vi "TemperatureLogger.vi"() -> ()   [LabVIEW 2022 SP3]
uses:
  <extravilib>/ChannelInstances/Tag-c(c(ref(LVObjVI()),bool),bool,bool,bool,path,u32,ref(UserDefinedRefnumTag))/Read With Abort.vi
  <extravilib>/ChannelInstances/Tag-c(c(ref(LVObjVI()),bool),bool,bool,bool,path,u32,ref(UserDefinedRefnumTag))/Write With Abort.vi
  <extravilib>/ChannelInstances/Tag-c(c(ref(LVObjVI()),bool),bool,bool,bool,path,u32,ref(UserDefinedRefnumTag))/Instantiate.vi
  <extravilib>/ChannelInstances/Tag-c(c(ref(LVObjVI()),bool),bool,bool,bool,path,u32,ref(UserDefinedRefnumTag))/EndpointRead.vi
  <vilib>/DAQmx/create/channels.llb/DAQmx Create Channel (AI-Temperature-Thermocouple).vi
  <extravilib>/ChannelInstances/Tag-c(c(ref(LVObjVI()),bool),bool,bool,bool,path,u32,ref(UserDefinedRefnumTag))/Endpoint.vi
  <extravilib>/ChannelInstances/Tag-c(c(ref(LVObjVI()),bool),bool,bool,bool,path,u32,ref(UserDefinedRefnumTag)).lvlib
panel:
  in  "NI Channel":tag
  in  "DAQmx Task":refnum<k21>
  in  "Thermc. Type":enum16{"J", "K", "N", "R", "S", "T", "B", "E"}(ring)
  in  "Start":bool
  out "Temperatures":dbl[][](graph)=[[1.25, 2.5, 3.7, 4.9], [1.25, 2.5, 3.7, 4.9], [1.25, 2.5, 3.7, 4.9], [1.25, 2.5, 3.7, 4.9], [1.25, 2.5, 3.7, 4.9], [1.25, 2.5, 3.7, 4.9], [1.25, 2.5, 3.7, 4.9], [1.25, 2.5, 3.7, 4.9], [1.25, 2.5, 3.7, 4.9], [1.25, 2.5, 3.7, 4.9], [1.25, 2.5, 3.7, 4.9], [1.25, 2.5, 3.7, 4.9], [1.25, 2.5, 3.7, 4.9], [1.25, 2.5, 3.7, 4.9], [1.25, 2.5, 3.7, 4.9], [1.25, 2.5, 3.7, 4.9], [1.25, 2.5, 3.7, 4.9], [1.25, 2.5, 3.7, 4.9], [1.25, 2.5, 3.7, 4.9], [1.25, 2.5, 3.7, 4.9], [1.25, 2.5, 3.7, 4.9], [1.25, 2.5, 3.7, 4.9], [1.25, 2.5, 3.7, 4.9], [1.25, 2.5, 3.7, 4.9], [1.25, 2.5, 3.7, 4.9], [1.25, 2.5, 3.7, 4.9], [1.25, 2.5, 3.7, 4.9], [1.25, 2.5, 3.7, 4.9], [1.25, 2.5, 3.7, 4.9], [1.25, 2.5, 3.7, 4.9], [1.25, 2.5, 3.7, 4.9], [1.25, 2.5, 3.7, 4.9], [1.25, 2.5, 3.7, 4.9], [1.25, 2.5, 3.7, 4.9], [1.25, 2.5, 3.7, 4.9], [1.25, 2.5, 3.7, 4.9], [1.25, 2.5, 3.7, 4.9], [1.25, 2.5, 3.7, 4.9], [1.25, 2.5, 3.7, 4.9], [1.25, 2.5, 3.7, 4.9], [1.25, 2.5, 3.7, 4.9], [1.25, 2.5, 3.7, 4.9], [1.25, 2.5, 3.7, 4.9], [1.25, 2.5, 3.7, 4.9], [1.25, 2.5, 3.7, 4.9], [1.25, 2.5, 3.7, 4.9], [1.25, 2.5, 3.7, 4.9], [1.25, 2.5, 3.7, 4.9]]
  out "String":string="Exiting"
  # "DAQmx Setup"
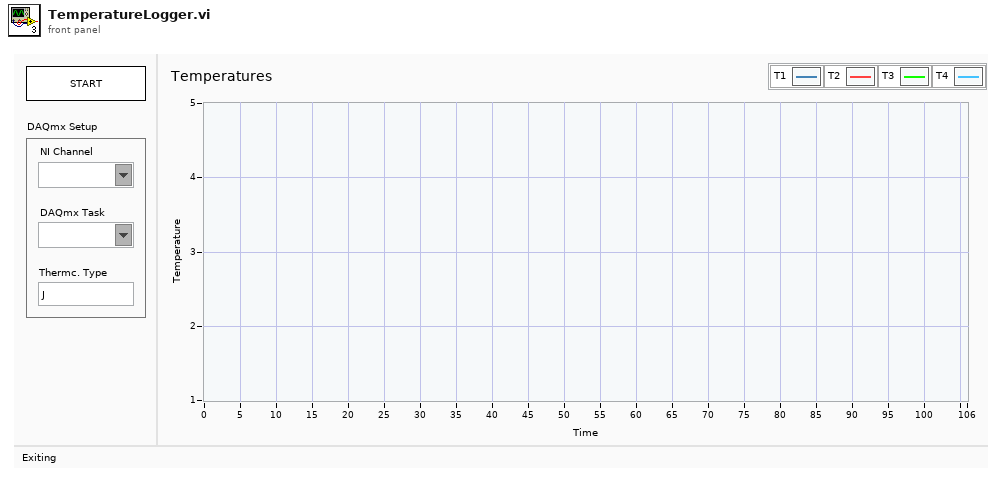
[diagram p1: front panel]
types:
  T1 = enum32{"Invalid", "Standard", "Closed", "Hidden", "Minimized", "Maximized"}
  T2 = enum32{"invalid app kind", "Development System", "Run Time System", "Student Edition", "Embedded LabVIEW", "Evaluation", "Custom"}
  T3 = cluster{"Core":cluster{"Current VI Reference":refnum<vi>, "Close Panel on Exit?":bool}, "System Active":bool, "Exit System":bool, "Connected":bool, "Data Path":path, "StartTime":u32, "NI Task":refnum<k21>}
  T4 = cluster{"Current VI Reference":refnum<vi>, "Close Panel on Exit?":bool}
  T5 = typedef "Tag-c(c(ref(LVObjVI()),bool),bool,bool,bool,path,u32,ref(UserDefinedRefnumTag)).lvlib/))Channel.ctl" = refnum<queue>
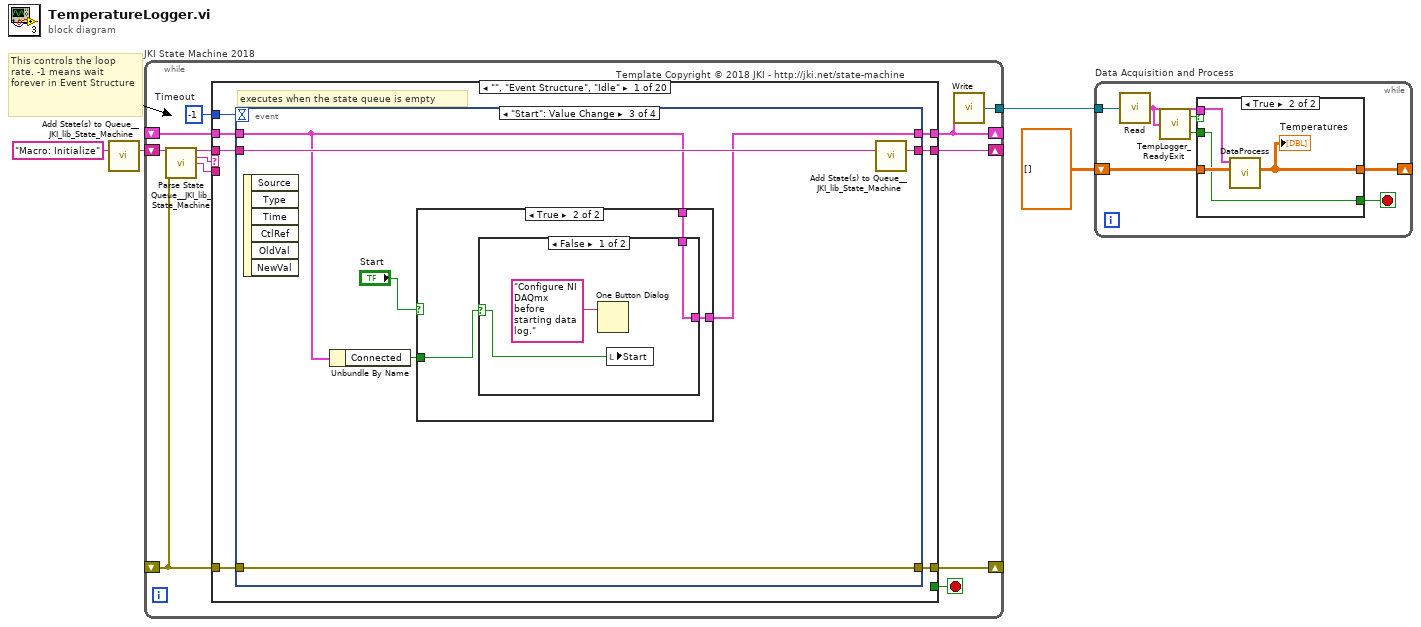
[diagram p0: block diagram]
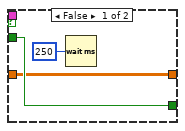
[diagram p2: hidden frame]
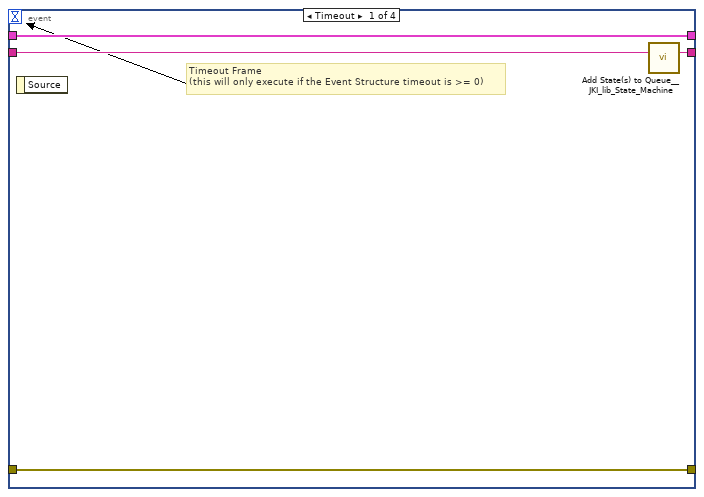
[diagram p3: hidden frame]
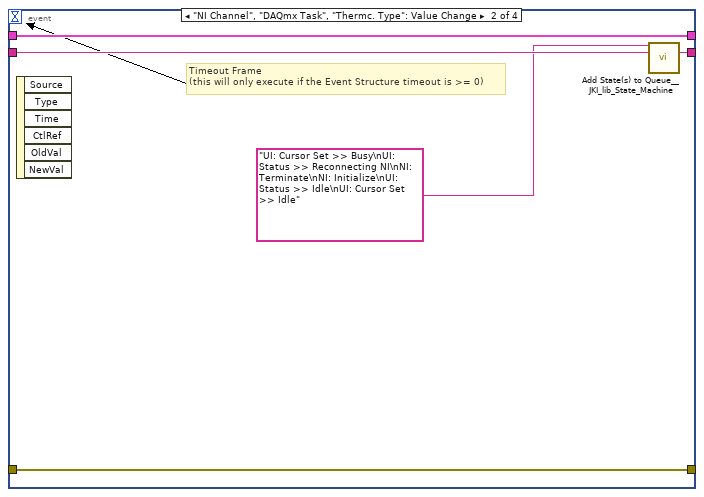
[diagram p4: hidden frame]
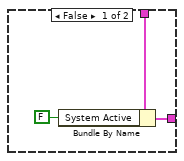
[diagram p5: hidden frame]
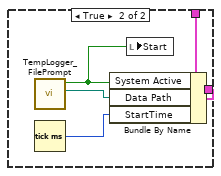
[diagram p6: hidden frame]
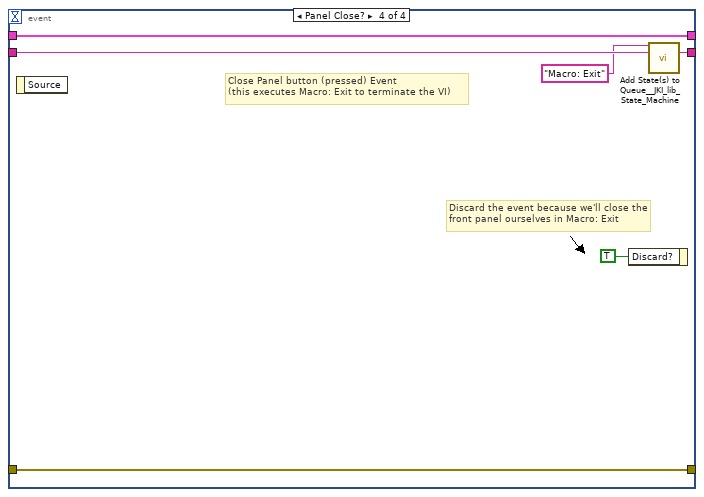
[diagram p7: hidden frame]
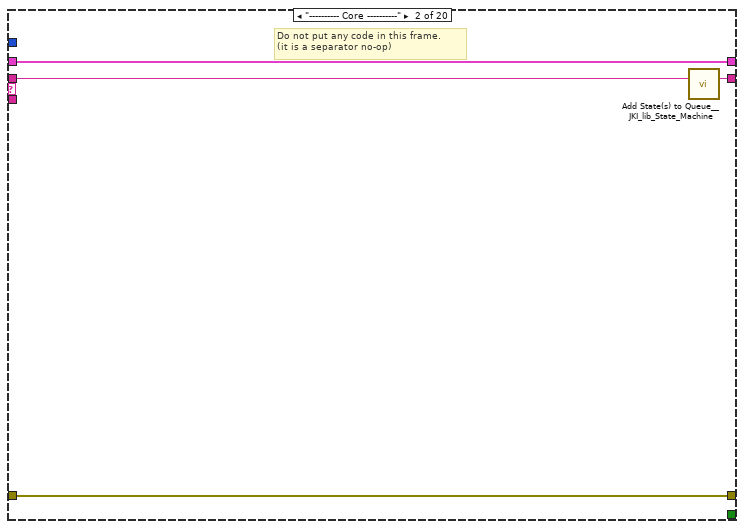
[diagram p8: hidden frame]
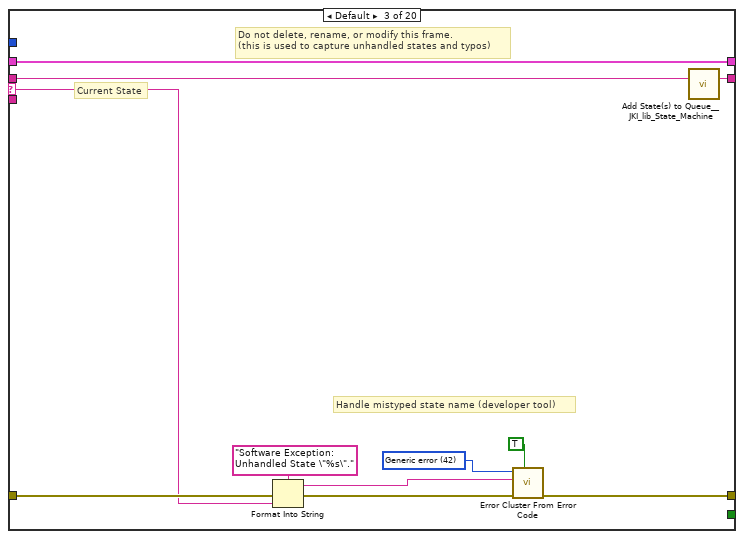
[diagram p9: hidden frame]
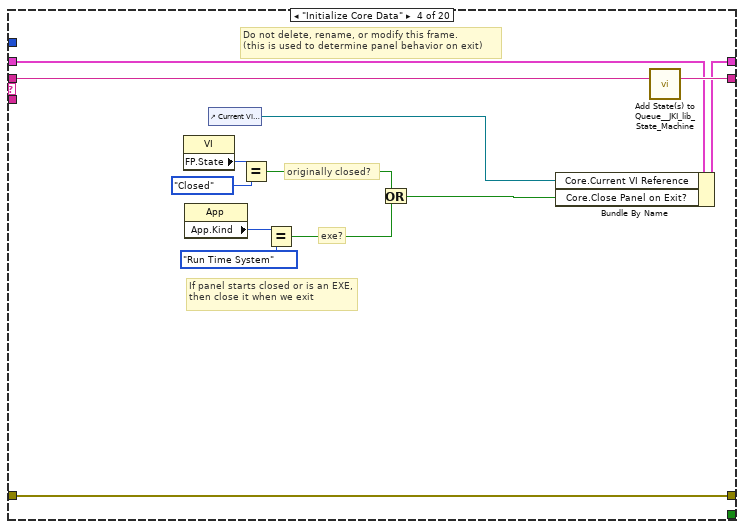
[diagram p10: hidden frame]
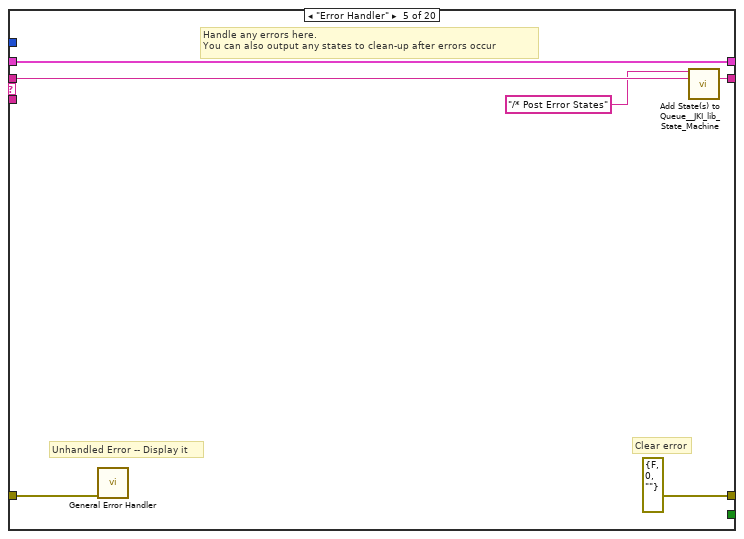
[diagram p11: hidden frame]
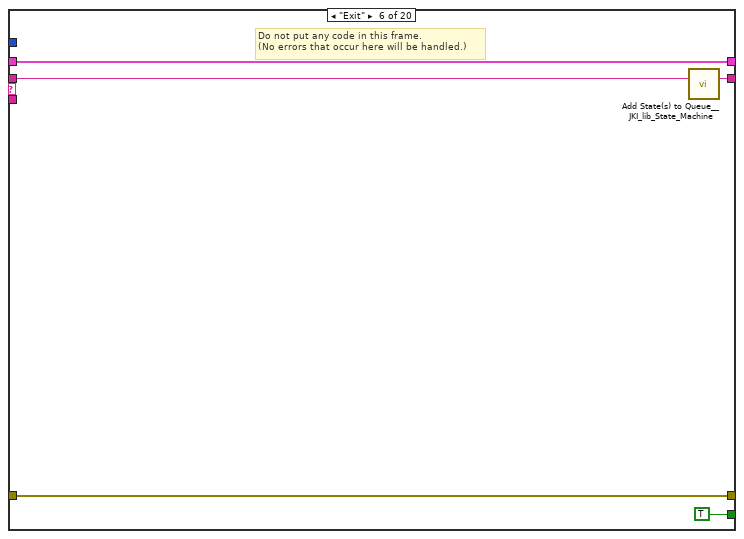
[diagram p12: hidden frame]
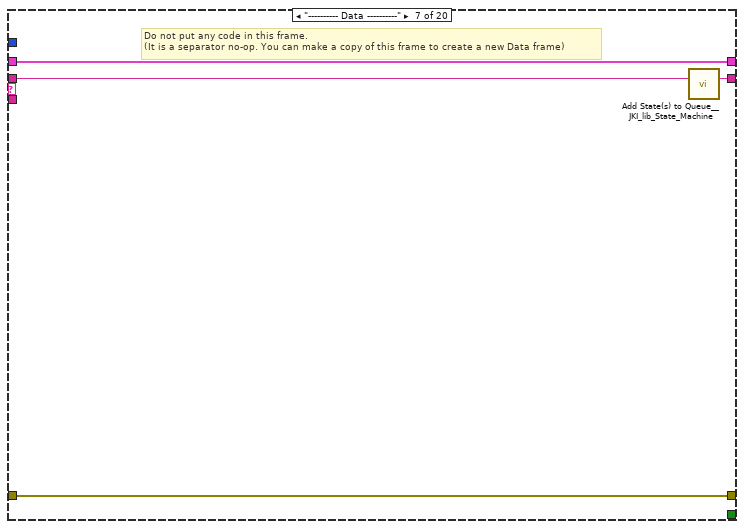
[diagram p13: hidden frame]
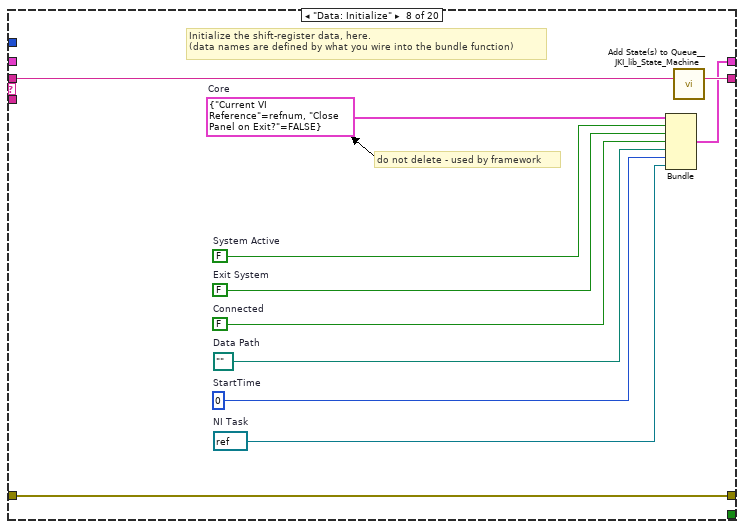
[diagram p14: hidden frame]
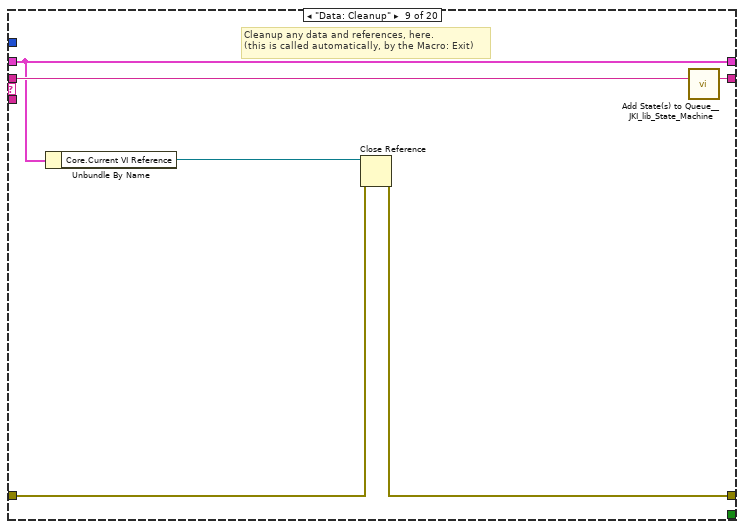
[diagram p15: hidden frame]
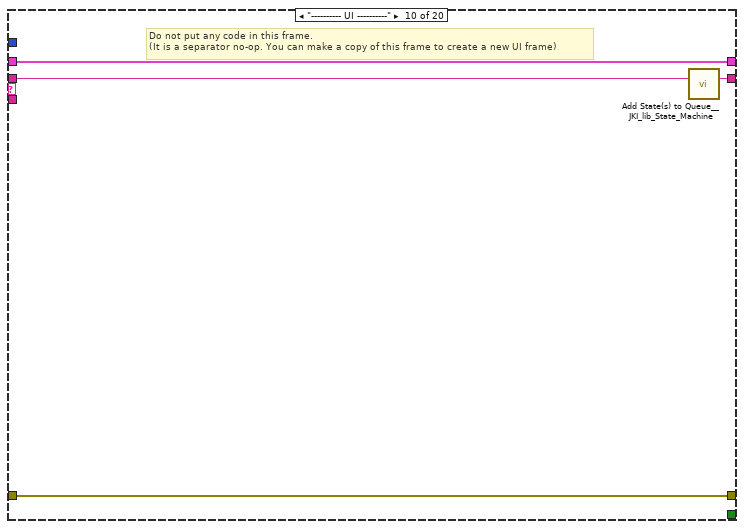
[diagram p16: hidden frame]
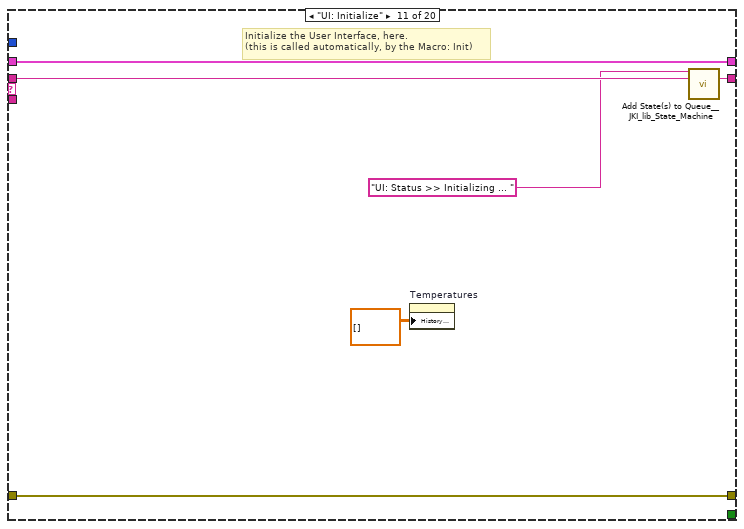
[diagram p17: hidden frame]
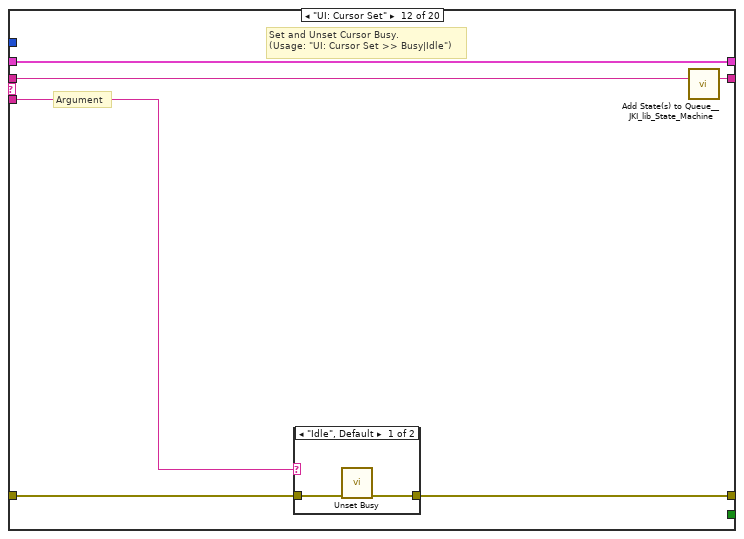
[diagram p18: hidden frame]
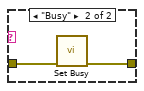
[diagram p19: hidden frame]
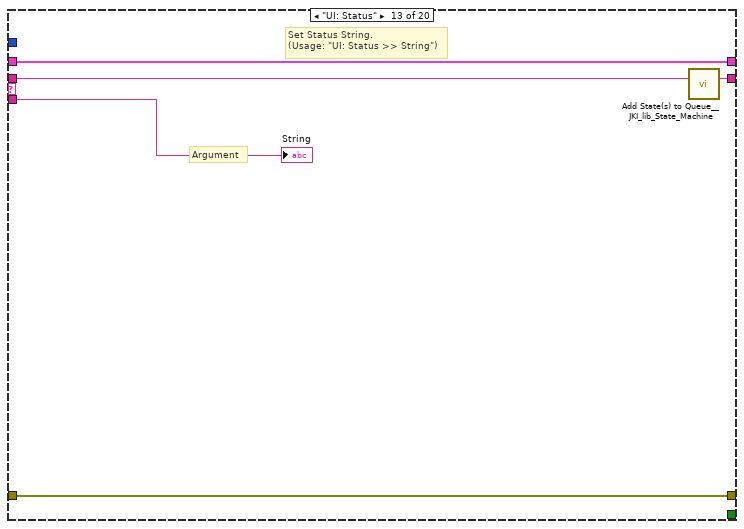
[diagram p20: hidden frame]
diagram:
  # "This controls the loop rate. -1 means wait forever in Event Structure"
  n1 = call <vilib>:"Add State(s) to Queue__JKI_lib_State_Machine.vi"("State(s) in (\"\")"="Macro: Initialize") -> ("States Out"=w4:string)  [unwired: 14 in]
  n2 = while "JKI State Machine 2018" {
    shift-right: [w6] -> _
    shift-left: _ -> [w9]
    shift-right: [w12] -> _
    shift-left: _ -> [w7]
    shift-right: [w11] -> _
    shift-left: w4 -> [w13]
    tunnel: [w5] -> w1
    stop <- w10 stop-if-true
    w8 = -1  # Timeout
    # "Template Copyright © 2018 JKI - http://jki.net/state-machine"
    n3 = call <vilib>:"Parse State Queue__JKI_lib_State_Machine.vi"("State Queue"=w13, "Error In (no error)"=w7) -> ("Remaining States"=w15:string, "Current State"=w16:string, "Arguments"=w14:string)  [unwired: 11 in]
    n4 = case shown="\"\", \"Event Structure\", \"Idle\"" w16 {
      selector: w16 -> [_ _ w64 _ _ _ _ _ _ _ _ _ _ _ _ _ _ _ _ _]
      tunnel: w15 -> [w23 w63 w68 w87 w93 w98 w102 w113 w119 w123 w129 w135 w144 w151 w220 w225 w237 w241 w253 w266]
      tunnel: w14 -> [_ _ _ _ _ _ _ _ _ _ _ w130 w141 w145 _ _ _ _ _ _]
      tunnel: w9 -> [w21 w60 w66 w80 w90 w96 w99 _ w114 w120 w127 w133 w142 w147 w217 w222 w234 w238 w250 w263]
      tunnel: [w20 w61 w70 w84 errorcluster {"status"=FALSE, "code"=0, "source"=""} ("error out") w95 w100 w110 w115 w121 w126 w131 w140 w148 w218 w223 w235 w239 w251 w264] -> w12
      tunnel: w7 -> [w19 w61 w69 w84 w89 w95 w100 w110 w116 w121 w126 w132 w140 w149 w218 w223 w235 w239 w251 w264]
      tunnel: [w22 w62 w67 w86 w92 w97 w101 w112 w118 w122 w128 w134 w143 w150 w219 w224 w236 w240 w252 w265] -> w11
      tunnel: [_ _ _ _ _ TRUE _ _ _ _ _ _ _ _ _ _ _ _ _ _] -> w10
      tunnel: [w18 w60 w66 w85 w90 w96 w99 w111 w114 w120 w127 w133 w142 w147 w217 w222 w227 w238 w244 w263] -> w6
      tunnel: w8 -> [w17 _ _ _ _ _ _ _ _ _ _ _ _ _ _ _ _ _ _ _]
      frame "", "Event Structure", "Idle" {
        # "executes when the state queue is empty"
        n5 = event shown="[2] \"Start\": Value Change" {
          selector: _ -> [_ _ _ _]
          dyn-events: _ -> [_ _ _ _]
          timeout: w17 -> [_ _ _ _]
          tunnel: w23 -> [w27 w32 w39 w59]
          tunnel: [w26 w31 w38 w58] -> w22
          tunnel: w21 -> [w24 w29 w34 w56]
          tunnel: [w25 w30 w37 w57] -> w20
          tunnel: w19 -> [w25 w30 w37 w57]
          tunnel: [w24 w29 w35 w56] -> w18
          event Timeout {
            # "Timeout Frame\n(this will only execute if the Event Structure timeout is >= 0)"
            n6 = event-data() -> ()  [unwired: 1 in, 1 out]
            n7 = call <vilib>:"Add State(s) to Queue__JKI_lib_State_Machine.vi"("State(s) in (\"\")"=w27) -> ("States Out"=w26:string)  [unwired: 14 in]
          }
          event "NI Channel", "DAQmx Task", "Thermc. Type": Value Change {
            # "Timeout Frame\n(this will only execute if the Event Structure timeout is >= 0)"
            n8 = event-data() -> ()  [unwired: 1 in, 6 out]
            n9 = call <vilib>:"Add State(s) to Queue__JKI_lib_State_Machine.vi"("State(s) in Front (\"\")"="UI: Cursor Set >> Busy\nUI: Status >> Reconnecting NI\nNI: Terminate\nNI: Initialize\nUI: Status >> Idle\nUI: Cursor Set >> Idle" ("State(s) in Front (\"\")"), "State(s) in (\"\")"=w32) -> ("States Out"=w31:string)  [unwired: 13 in]
          }
          event "Start": Value Change {
            n10 = event-data() -> ()  [unwired: 1 in, 6 out]
            n11 = Unbundle By Name(w34) -> ("Connected"=w33:bool)
            n12 = case shown="True" "Start" {
              tunnel: w34 -> [w40 w45]
              tunnel: [w41 w44] -> w35
              tunnel: w33 -> [_ w43]
              frame False {
                n13 = Bundle By Name(cluster=w40, "System Active"=FALSE) -> (w41:T3)
              }
              frame True {
                n14 = case shown="False" w43 {
                  selector: w43 -> [w46 _]
                  tunnel: w45 -> [w47 w53]
                  tunnel: [w47 w52] -> w44
                  frame False {
                    n15 = One Button Dialog(message="Configure NI DAQmx before starting data log.") -> ()  [unwired: 1 in, 1 out]
                    n16 = local write "Start"(w46) -> ()
                  }
                  frame True {
                    n17 = call "TempLogger_FilePrompt.vi"() -> ("selected path"=w51:path, "not cancelled"=w50:bool)  [unwired: 10 in]
                    n18 = Tick Count (ms)() -> (millisecond timer value=w49:u32)
                    n19 = Bundle By Name(cluster=w53, "System Active"=w50, "Data Path"=w51, "StartTime"=w49) -> (w52:T3)
                    n20 = local write "Start"(w50) -> ()
                  }
                }
              }
            }
            n21 = call <vilib>:"Add State(s) to Queue__JKI_lib_State_Machine.vi"("State(s) in (\"\")"=w39) -> ("States Out"=w38:string)  [unwired: 14 in]
          }
          event Panel Close? {
            # "Discard the event because we'll close the front panel ourselves in Macro: Exit"
            # "Close Panel button (pressed) Event\n(this executes Macro: Exit to terminate the VI)"
            n22 = event-data() -> ()  [unwired: 1 in, 1 out]
            n23 = event-data("Discard?"=TRUE) -> ()  [unwired: 1 in, 1 out]
            n24 = call <vilib>:"Add State(s) to Queue__JKI_lib_State_Machine.vi"("State(s) in Front (\"\")"="Macro: Exit", "State(s) in (\"\")"=w59) -> ("States Out"=w58:string)  [unwired: 13 in]
          }
        }
      }
      frame "---------- Core ----------" {
        # "Do not put any code in this frame.\n(it is a separator no-op)"
        n25 = call <vilib>:"Add State(s) to Queue__JKI_lib_State_Machine.vi"("State(s) in (\"\")"=w63) -> ("States Out"=w62:string)  [unwired: 14 in]
      }
      frame Default {
        w73 = 42 items=["No error", "Argument error", "Memory is full", "Out of zone", "End of file", "File already open", "Generic file I/O error", "File not found", "File permission error", "Disk is full", "Duplicate path", "Too many files open", "System feature not enabled", "Resource file not found", "Cannot add resource", "Resource not found", "Image not found", "Image memory error", "Pen does not exist", "Config type invalid", "Config token not found", "Config parse error", "Config memory error", "Bad external code format", "Bad external code offset", "External code not present", "Null window", "Destroy window error", "Null menu", "Print aborted", "Bad print record", "Print driver error", "Windows error during printing", "Memory error during printing", "Print dialog error", "Generic print error", "Invalid device refnum", "Device not found", "Device parameter error", "Device unit error", "Cannot open device", "Device call aborted", "Generic error", "Cancelled by user", "Object ID too low", "Object ID too high", "Object not in heap", "Unknown heap", "Unknown object (invalid DefProc)", "Unknown object (DefProc not in table)", "Message out of range", "Invalid (null) method", "Unknown message", "Manager call not supported", "Bad address", "Network operation in progress", "Network operation timed out", "Connection is busy", "Network attribute not supported", "Network error", "Address in use", "System out of memory", "Connection aborted", "Connection refused", "Not connected", "Already connected", "Connection closed", "Initialization error (interapplication manager)", "Bad occurrence", "Wait on unbound occurrence handler", "Occurrence queue overflow", "Datalog type conflict", "Unused", "Unrecognized type (interapplication manager)", "Memory corrupt", "Failed to make temporary DLL", "Old CIN version", "Drag socket not found", "Failed to load drop-object", "Failed to register OLE object", "Failed to release OLE object", "Format specifier type mismatch", "Unknown format specifier", "Too few format specifiers", "Too many format specifiers", "Scan failed", "Newer CIN version", "Error converting to variant", "Runtime menu error", "Password tampered", "Variant attribute not found", "Incompatible variant data type", "Event data is not available", "Event Store is not present", "Occurrence is not found", "Event Queue is not created", "Event info is not available", "Refnum passed is NULL", "Error retrieving Class GUID", "Error retrieving CoClass GUID", "Error retrieving TypeLib GUID.", "Bad built application magic bytes.", "Specific driver is different from the specific driver associated with the Logical Name.", "There is no session opened to the class driver.", "Max Error", "MAX - Error with config objects", "MAX - Error loading configuration", "MAX - Group not supported"]
        # "Current State"
        # "Do not delete, rename, or modify this frame.\n(this is used to capture unhandled states and typos)"
        # "Handle mistyped state name (developer tool)"
        n26 = Format Into String(format string="Software Exception: Unhandled State \"%s\"." ("message"), error in=w69, w64) -> (resulting string=w72:string, error out=w71:errorcluster)  [unwired: 1 in]
        n27 = call <vilib>:"Error Cluster From Error Code.vi"("show call chain? (False)"=TRUE, "error in (no error)"=w71, "error message (\"\")"=w72, "error code (0)"=w73) -> ("error out"=w70:errorcluster)  [unwired: 5 in]
        n28 = call <vilib>:"Add State(s) to Queue__JKI_lib_State_Machine.vi"("State(s) in (\"\")"=w68) -> ("States Out"=w67:string)  [unwired: 14 in]
      }
      frame "Initialize Core Data" {
        # "Do not delete, rename, or modify this frame.\n(this is used to determine panel behavior on exit)"
        # "originally closed?"
        # "exe?"
        # "If panel starts closed or is an EXE, then close it when we exit"
        n29 = property class="VI"() -> ("FP.State"=w77:T1)  [unwired: 2 in, 2 out]
        n30 = property class="App"() -> ("App.Kind"=w83:T2)  [unwired: 2 in, 2 out]
        n31 = control-ref of="Current VI Reference"() -> (w78:refnum<vi>)
        n32 = Equal?(x=w77, y=T1."Closed" ("Front Panel Window:State")) -> (x = y?=w75:bool)
        n33 = Equal?(x=w83, y=T2."Run Time System" ("Application:Kind")) -> (x = y?=w81:bool)
        n34 = Or(x=w75, y=w81) -> (x .or. y?=w79:bool)
        n35 = Bundle By Name(cluster=w80, "Core.Current VI Reference"=w78, "Core.Close Panel on Exit?"=w79) -> (w85:T3)
        n36 = call <vilib>:"Add State(s) to Queue__JKI_lib_State_Machine.vi"("State(s) in (\"\")"=w87) -> ("States Out"=w86:string)  [unwired: 14 in]
      }
      frame "Error Handler" {
        # "Unhandled Error -- Display it"
        # "Handle any errors here.\nYou can also output any states to clean-up after errors occur"
        # "Clear error"
        n37 = call <vilib>:"General Error Handler.vi"("error in (no error)"=w89) -> ()  [unwired: 10 in, 5 out]
        n38 = call <vilib>:"Add State(s) to Queue__JKI_lib_State_Machine.vi"("State(s) in Front (\"\")"="/* Post Error States", "State(s) in (\"\")"=w93) -> ("States Out"=w92:string)  [unwired: 13 in]
      }
      frame "Exit" {
        # "Do not put any code in this frame.\n(No errors that occur here will be handled.)"
        n39 = call <vilib>:"Add State(s) to Queue__JKI_lib_State_Machine.vi"("State(s) in (\"\")"=w98) -> ("States Out"=w97:string)  [unwired: 14 in]
      }
      frame "---------- Data ----------" {
        # "Do not put any code in this frame.\n(It is a separator no-op. You can make a copy of this frame to create a new Data frame)"
        n40 = call <vilib>:"Add State(s) to Queue__JKI_lib_State_Machine.vi"("State(s) in (\"\")"=w102) -> ("States Out"=w101:string)  [unwired: 14 in]
      }
      frame "Data: Initialize" {
        w103 = refnum<k21> refnum  # NI Task
        w104 = FALSE  # Connected
        w105 = u32 0  # StartTime
        w106 = path ""  # Data Path
        w107 = FALSE  # Exit System
        w108 = T4 {"Current VI Reference"=refnum, "Close Panel on Exit?"=FALSE}  # Core
        w109 = FALSE  # System Active
        # "do not delete - used by framework"
        # "Initialize the shift-register data, here.\n(data names are defined by what you wire into the bundle function)"
        n41 = Bundle("Core"=w108, "System Active"=w109, "Exit System"=w107, "Connected"=w104, "Data Path"=w106, "StartTime"=w105, "NI Task"=w103) -> (w111:T3)  [unwired: 1 in]
        n42 = call <vilib>:"Add State(s) to Queue__JKI_lib_State_Machine.vi"("State(s) in (\"\")"=w113) -> ("States Out"=w112:string)  [unwired: 14 in]
      }
      frame "Data: Cleanup" {
        # "Cleanup any data and references, here.\n(this is called automatically, by the Macro: Exit)"
        n43 = Unbundle By Name(w114) -> ("Core.Current VI Reference"=w117:refnum<vi>)
        n44 = Close Reference(reference=w117, error in (no error)=w116) -> (error out=w115:errorcluster)
        n45 = call <vilib>:"Add State(s) to Queue__JKI_lib_State_Machine.vi"("State(s) in (\"\")"=w119) -> ("States Out"=w118:string)  [unwired: 14 in]
      }
      frame "---------- UI ----------" {
        # "Do not put any code in this frame.\n(It is a separator no-op. You can make a copy of this frame to create a new UI frame)"
        n46 = call <vilib>:"Add State(s) to Queue__JKI_lib_State_Machine.vi"("State(s) in (\"\")"=w123) -> ("States Out"=w122:string)  [unwired: 14 in]
      }
      frame "UI: Initialize" {
        # "Initialize the User Interface, here.\n(this is called automatically, by the Macro: Init)"
        n47 = property on="Temperatures" class="WFChart (strict)"("History Data"=dbl[][] []) -> ()  [unwired: 2 in, 2 out]
        n48 = call <vilib>:"Add State(s) to Queue__JKI_lib_State_Machine.vi"("State(s) in Front (\"\")"="UI: Status >> Initializing ... " ("State(s) in Front (\"\")"), "State(s) in (\"\")"=w129) -> ("States Out"=w128:string)  [unwired: 13 in]
      }
      frame "UI: Cursor Set" {
        # "Argument"
        # "Set and Unset Cursor Busy.\n(Usage: \"UI: Cursor Set >> Busy|Idle\")"
        n49 = case shown="\"Idle\", Default" w130 {
          tunnel: w132 -> [w137 w139]
          tunnel: [w136 w138] -> w131
          frame "Idle", Default {
            n50 = call <vilib>:"Unset Busy.vi"("error in (no error)"=w137) -> ("error out"=w136:errorcluster)  [unwired: 10 in]
          }
          frame "Busy" {
            n51 = call <vilib>:"Set Busy.vi"("error in (no error)"=w139) -> ("error out"=w138:errorcluster)  [unwired: 9 in, 1 out]
          }
        }
        n52 = call <vilib>:"Add State(s) to Queue__JKI_lib_State_Machine.vi"("State(s) in (\"\")"=w135) -> ("States Out"=w134:string)  [unwired: 14 in]
      }
      frame "UI: Status" {
        # "Argument"
        # "Set Status String.\n(Usage: \"UI: Status >> String\")"
        n53 = call <vilib>:"Add State(s) to Queue__JKI_lib_State_Machine.vi"("State(s) in (\"\")"=w144) -> ("States Out"=w143:string)  [unwired: 14 in]
        "String" <- w141
      }
      frame "UI: Front Panel State" {
        # "Argument"
        # "Set Front Panel Open or Closed\n(Usage: \"UI: Front Panel State >> Open|Close\")"
        n54 = Unbundle By Name(w147) -> ("Core.Current VI Reference"=w146:refnum<vi>)
        n55 = case shown="\"Hidden\", \"Hide\"" w145 {
          tunnel: w149 -> [w157 w172 w183 w196 w209]
          tunnel: [w159 w173 w185 w198 w211] -> w148
          tunnel: w146 -> [w158 w170 w184 w197 w210]
          frame "Open", "Standard", Default {
            w152 = T1."Standard" ("State")
            n56 = property class="VI"(reference=w158, error in=w157) -> (reference out=w155:refnum<vi>, error out=w156:errorcluster, "FP.State"=w154:T1)
            n57 = Not Equal?(x=w154, y=w152) -> (x != y?=w153:bool)
            n58 = case shown="True" w153 {
              tunnel: [w163 w165] -> w159
              tunnel: w156 -> [w162 w165]
              tunnel: w155 -> [w161 _]
              tunnel: w152 -> [w160 _]
              frame True {
                n59 = invoke class="VI" method="FP.Open"(reference=w161, error in=w162, "Activate"=TRUE, "State"=w160) -> (error out=w163:errorcluster)  [unwired: 1 in, 4 out]
              }
              frame False {
              }
            }
          }
          frame "Close", "Closed" {
            n60 = property class="VI"(reference=w170, error in=w172) -> (reference out=w169:refnum<vi>, error out=w171:errorcluster, "FP.State"=w167:T1)
            n61 = Not Equal?(x=w167, y=T1."Closed" ("Front Panel Window:State")) -> (x != y?=w166:bool)
            n62 = case shown="True" w166 {
              tunnel: [w174 w177] -> w173
              tunnel: w171 -> [w174 w176]
              tunnel: w169 -> [_ w175]
              frame False {
              }
              frame True {
                n63 = invoke class="VI" method="FP.Close"(reference=w175, error in=w176) -> (error out=w177:errorcluster)  [unwired: 1 in, 2 out]
              }
            }
          }
          frame "Hidden", "Hide" {
            w178 = T1."Hidden" ("State")
            n64 = property class="VI"(reference=w184, error in=w183) -> (reference out=w181:refnum<vi>, error out=w182:errorcluster, "FP.State"=w180:T1)
            n65 = Not Equal?(x=w180, y=w178) -> (x != y?=w179:bool)
            n66 = case shown="True" w179 {
              tunnel: [w189 w190] -> w185
              tunnel: w182 -> [w188 w190]
              tunnel: w181 -> [w187 _]
              tunnel: w178 -> [w186 _]
              frame True {
                n67 = invoke class="VI" method="FP.Open"(reference=w187, error in=w188, "State"=w186) -> (error out=w189:errorcluster)  [unwired: 2 in, 4 out]
              }
              frame False {
              }
            }
          }
          frame "Minimize", "Minimized" {
            w191 = T1."Minimized" ("State")
            n68 = property class="VI"(reference=w197, error in=w196) -> (reference out=w194:refnum<vi>, error out=w195:errorcluster, "FP.State"=w193:T1)
            n69 = Not Equal?(x=w193, y=w191) -> (x != y?=w192:bool)
            n70 = case shown="True" w192 {
              tunnel: [w202 w203] -> w198
              tunnel: w195 -> [w201 w203]
              tunnel: w194 -> [w200 _]
              tunnel: w191 -> [w199 _]
              frame True {
                n71 = invoke class="VI" method="FP.Open"(reference=w200, error in=w201, "State"=w199) -> (error out=w202:errorcluster)  [unwired: 2 in, 4 out]
              }
              frame False {
              }
            }
          }
          frame "Maximize", "Maximized" {
            w204 = T1."Maximized" ("State")
            n72 = property class="VI"(reference=w210, error in=w209) -> (reference out=w207:refnum<vi>, error out=w208:errorcluster, "FP.State"=w206:T1)
            n73 = Not Equal?(x=w206, y=w204) -> (x != y?=w205:bool)
            n74 = case shown="True" w205 {
              tunnel: [w215 w216] -> w211
              tunnel: w208 -> [w214 w216]
              tunnel: w207 -> [w213 _]
              tunnel: w204 -> [w212 _]
              frame True {
                n75 = invoke class="VI" method="FP.Open"(reference=w213, error in=w214, "State"=w212) -> (error out=w215:errorcluster)  [unwired: 2 in, 4 out]
              }
              frame False {
              }
            }
          }
        }
        n76 = call <vilib>:"Add State(s) to Queue__JKI_lib_State_Machine.vi"("State(s) in (\"\")"=w151) -> ("States Out"=w150:string)  [unwired: 14 in]
      }
      frame "---------- Macro ----------" {
        # "Do not put any code in this frame.\n(It is a separator no-op. You can make a copy of this frame to create a new Macro frame)"
        n77 = call <vilib>:"Add State(s) to Queue__JKI_lib_State_Machine.vi"("State(s) in (\"\")"=w220) -> ("States Out"=w219:string)  [unwired: 14 in]
      }
      frame "Macro: Initialize" {
        w221 = "Data: Initialize\nInitialize Core Data\nUI: Initialize\nUI: Front Panel State >> Open\nUI: Cursor Set >> Busy\nUI: Status >> Connecting NI\nNI: Initialize\nUI: Status >> Idle\nUI: Cursor Set >> Idle"  # Data: Initialize Initialize Core Data UI: Initialize UI: Front Panel State >> Open UI: Cursor Set >> Busy UI: Status >> Connecting NI NI: Initialize UI: Status >> Idle UI: Cursor Set >> Idle
        # "Initialization Macro\n(This is called once, when the VI starts)"
        n78 = call <vilib>:"Add State(s) to Queue__JKI_lib_State_Machine.vi"("State(s) in Front (\"\")"=w221, "State(s) in (\"\")"=w225) -> ("States Out"=w224:string)  [unwired: 13 in]
      }
      frame "Macro: Exit" {
        # "Exit Macro\n(This is called once, when the VI exits)"
        n79 = Unbundle By Name(w234) -> ("Core.Close Panel on Exit?"=w233:bool)
        n80 = Bundle By Name(cluster=w234, "Exit System"=TRUE) -> (w227:T3)
        n81 = Select(t="UI: Front Panel State >> Close", s=w233, f="") -> (s? t:f=w230:string)
        n82 = call <vilib>:"Add State(s) to Queue__JKI_lib_State_Machine.vi"("State(s) in (\"\")"=w230, "State(s) at Back (\"\")"="UI: Cursor Set >> Busy\nUI: Status >> Cleaning Data\nData: Cleanup\nUI: Status >> Teminating NI Connection\nNI: Terminate\nUI: Status >> Exiting\nUI: Cursor Set >> Idle\nExit") -> ("States Out"=w228:string)  [unwired: 13 in]
        n83 = call <vilib>:"Add State(s) to Queue__JKI_lib_State_Machine.vi"("State(s) in Front (\"\")"=w228, "State(s) in (\"\")"=w237) -> ("States Out"=w236:string)  [unwired: 13 in]
      }
      frame "---------- NI ----------" {
        # "Template Separator\n(You can make a copy of, or modify, this frame)"
        n84 = call <vilib>:"Add State(s) to Queue__JKI_lib_State_Machine.vi"("State(s) in (\"\")"=w241) -> ("States Out"=w240:string)  [unwired: 14 in]
      }
      frame "NI: Initialize" {
        # "Your code here.\n(You can make a copy of, or modify, this frame)"
        n85 = call-poly <vilib>:"DAQmx Create Virtual Channel.vi"("task in"="DAQmx Task", "physical channels"="NI Channel", "thermocouple type"="Thermc. Type") -> ("task out"=w249:refnum<k21>, "error out"=w248:errorcluster)  [unwired: 11 in]
        n86 = call <vilib>:"DAQmx Start Task.vi"("task/channels in"=w249, "error in"=w248) -> ("task out"=w242:refnum<k21>, "error out"=w243:errorcluster)  [unwired: 12 in]
        n87 = case shown="No Error" w243 {
          tunnel: w250 -> [w257 w260]
          tunnel: [w255 w259] -> w244
          tunnel: w242 -> [w254 _]
          frame No Error {
            n88 = Bundle By Name(cluster=w257, "NI Task"=w254, "Connected"=TRUE) -> (w255:T3)
          }
          frame Error {
            n89 = Bundle By Name(cluster=w260, "Connected"=FALSE) -> (w259:T3)
          }
        }
        n90 = call <vilib>:"Add State(s) to Queue__JKI_lib_State_Machine.vi"("State(s) in (\"\")"=w253) -> ("States Out"=w252:string)  [unwired: 14 in]
      }
      frame "NI: Terminate" {
        # "Your code here.\n(You can make a copy of, or modify, this frame)"
        n91 = Unbundle By Name(w263) -> ("NI Task"=w262:refnum<k21>, "Connected"=w261:bool)
        n92 = case shown="False" w261 {
          tunnel: w262 -> [_ w267]
          frame False {
          }
          frame True {
            n93 = call <vilib>:"DAQmx Stop Task.vi"("task/channels in"=w267) -> ()  [unwired: 13 in, 2 out]
          }
        }
        n94 = call <vilib>:"Add State(s) to Queue__JKI_lib_State_Machine.vi"("State(s) in (\"\")"=w266) -> ("States Out"=w265:string)  [unwired: 14 in]
      }
    }
    n95 = call <extravilib>:"Write.vi"("element"=w6) -> ("channel"=w5:T5)  [unwired: 1 out]
  }
  n96 = while "Data Acquisition and Process" {
    shift-right: [w271] -> _
    shift-left: dbl[][] [] -> [w274]
    tunnel: w1 -> [w273]
    stop <- w272 stop-if-true
    n97 = call <extravilib>:"Read.vi"("channel"=w273) -> ("element"=w270:T3)  [unwired: 1 in, 1 out]
    n98 = call "TempLogger_ReadyExit.vi"("element"=w270) -> ("Connected"=w268:bool, "Exit System"=w269:bool)
    n99 = case shown="True" w268 {
      tunnel: w274 -> [w275 w281]
      tunnel: [w276 w278] -> w272
      tunnel: [w275 w280] -> w271
      tunnel: w270 -> [_ w279]
      tunnel: w269 -> [w276 w278]
      frame False {
        n100 = Wait (ms)(milliseconds to wait=u32 250) -> ()  [unwired: 1 out]
      }
      frame True {
        n101 = call "DataProcess.vi"("Data in"=w281, "element"=w279) -> ("Data out"=w280:dbl[][])  [unwired: 8 in, 1 out]
        "Temperatures" <- w280
      }
    }
  }
